vi "Read ImageJ Import File.vi"(8 "error in":errorcluster, 11 "Path In":path) -> (0 "error IO":errorcluster, 2 "Raw File Params":cluster{"raw offset":u32, "raw frame gap":u32}, 3 "Path Out":path)   [LabVIEW 2023, in "Photometrics Camera.lvlib"]
uses:
  Photometrics Camera.lvlib
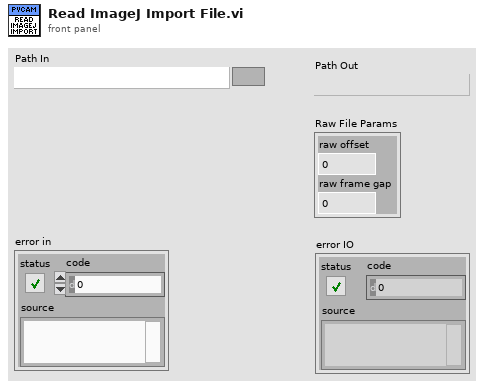
[diagram p1: front panel]
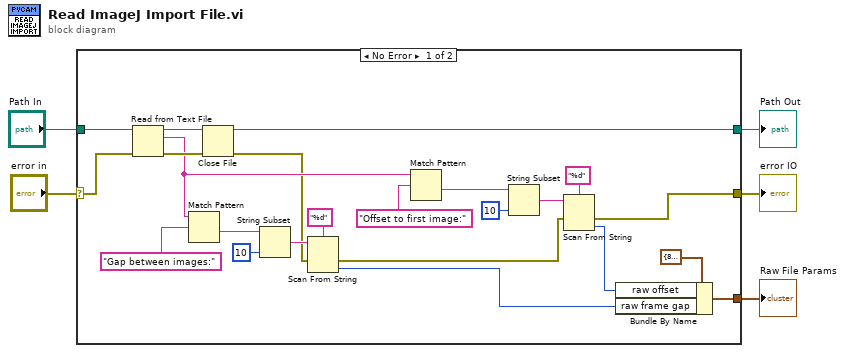
[diagram p0: block diagram]
diagram:
  n1 = case shown="No Error" "error in" {
    selector: "error in" -> [w25 w30]
    tunnel: "Path In" -> [w26 w29]
    tunnel: [w6 w30] -> w3
    tunnel: [w24 w29] -> w2
    tunnel: [w9 _] -> w1
    frame No Error {
      n2 = Read from Text File(file (use dialog)=w26, error in=w25) -> (refnum out=w27:refnum<file>, text=w23:string, error out=w28:errorcluster)  [unwired: 2 in, 1 out]
      n3 = Match Pattern(string=w23, regular expression="Gap between images:") -> (after substring=w20:string)  [unwired: 1 in, 3 out]
      n4 = Close File(refnum=w27, error in=w28) -> (path=w24:path, error out=w7:errorcluster)
      n5 = String Subset(string=w20, length (rest)=10 ("length (rest)")) -> (substring=w18:string)  [unwired: 1 in]
      n6 = Scan From String(format string="%d", input string=w18, error in=w7) -> (error out=w8:errorcluster, output 1=w10:i32)  [unwired: 2 in, 2 out]
      n7 = Match Pattern(string=w23, regular expression="Offset to first image:") -> (after substring=w13:string)  [unwired: 1 in, 3 out]
      n8 = String Subset(string=w13, length (rest)=10 ("length (rest)")) -> (substring=w15:string)  [unwired: 1 in]
      n9 = Scan From String(format string="%d", input string=w15, error in=w8) -> (error out=w6:errorcluster, output 1=w11:i32)  [unwired: 2 in, 2 out]
      n10 = Bundle By Name(cluster=cluster{"raw offset":u32, "raw frame gap":u32} {"raw offset"=80, "raw frame gap"=4096}, "raw offset"=w11, "raw frame gap"=w10) -> (w9:cluster{"raw offset":u32, "raw frame gap":u32})
    }
    frame Error {
    }
  }
  "error IO" <- w3
  "Path Out" <- w2
  "Raw File Params" <- w1
